vi "read.vi"(8 "error in (no error)":errorcluster, 11 "MKS in":refnum<class "MKS.lvclass">) -> (0 "error out":errorcluster, 2 "Data":dbl[](array[numeric]), 3 "MKS out":refnum<class "MKS.lvclass">)   [LabVIEW 2022 SP3, in "MKS.lvclass"]
uses:
  MKS.lvclass
  MKS.lvclass/MKS.ctl
  <instrlib>/MKS 972B/MKS 972B.lvlib
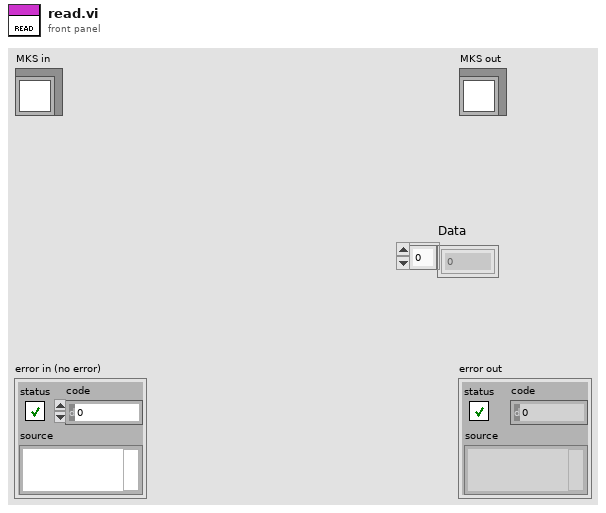
[diagram p1: front panel]
types:
  T1 = typedef "MKS 972B.lvlib/Unit address.ctl" = u32
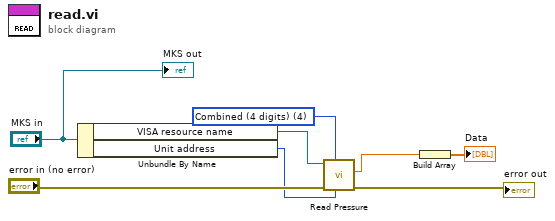
[diagram p0: block diagram]
diagram:
  w5 = u16 4 items=["MicroPirani value (3 digits)"=1, "Cold Cathode value (3 digits)"=2, "Combined (3 digits)"=3, "Combined (4 digits)"=4] ("Reading mode")
  n1 = Unbundle By Name("MKS in") -> ("VISA resource name"=w8:refnum<visa-resource-name>, "Unit address"=w6:T1)
  n2 = call <instrlib>:"Read Pressure.vi"("Unit address (001-253)"=w6, "Reading mode"=w5, "error in (no error)"="error in (no error)", "VISA resource name"=w8) -> ("error out"=→"error out":errorcluster, "Pressure value"=w3:dbl)  [unwired: 5 in, 1 out]
  n3 = Build Array(w3) -> (→"Data":dbl[])
  "MKS out" <- "MKS in"
